vi "navX Close.vi"(8 "error in (no error)":errorcluster, 11 "navX Device TypeDef":T1={"navX Interface Protocol"=enum."SPI", "navX Interface Protocol TypeDefs"={"SPIDevRef"={"DevStatus"={"status"=FALSE, "code"=0, "source"=""}, "Handle"=0, "Controller"=enum."Controller 1", "SPI Bus"=enum."SPI On-Board, CS0"}, "I2CDevRef"={"DevStatus"={"status"=FALSE, "code"=0, "source"=""}, "Controller"=enum."Controller 1", "Device Address"=0, "Handle"=0, "I2C Bus"=enum."Invalid"}}, "navX System Information"={"Board Information"={"WhoAmI (50 | 0x32)"=0, "Board Revision"=0, "Firmware Major Version"=0, "Firmware Minor Version"=0}, "Status"={"Update Rate Hz"=0, "Accelerometer Full-Scale Range"=0, "Gyro Full-Scale Range"=0, "NAVX_OP_STATUS"=0, "NAVX_CAL_STATUS"=0, "NAVX_SELFTEST_STATUS"=0, "NAVX_SENSOR_STATUS"={"MOVING"=FALSE, "YAW_STABLE"=FALSE, "MAG_DISTURBANCE"=FALSE, "ALTITUDE_VALID"=FALSE, "SEALEVEL_PRESS_SET"=FALSE, "FUSED_HEADING_VALID"=FALSE}}, "Offsets"={"Yaw"=0.0, "Quat W"=0.0, "Quat X"=0.0, "Quat Y"=0.0, "Quat Z"=0.0}}, "navX Common Information"={"Update Rate (4Hz-60Hz)"=50, "refnum name"="", "error"={"status"=FALSE, "code"=0, "source"=""}}} {"navX Common Information"."Update Rate (4Hz-60Hz)" min=4 max=50 step=1; "navX System Information"."Status"."NAVX_OP_STATUS" items=["INITIALIZING", "SELFTEST_IN_PROGRESS", "ERROR", "IMU_AUTOCAL_IN_PROGRESS", "NORMAL"]; "navX System Information"."Status"."NAVX_CAL_STATUS" items=["IMU_CAL_STATE_MASK"=3, "IMU_CAL_INPROGRESS"=0, "IMU_CAL_ACCUMULATE"=1, "IMU_CAL_COMPLETE"=2, "MAG_CAL_COMPLETE"=4, "BARO_CAL_COMPLETE"=8]; "navX Interface Protocol TypeDefs"."I2CDevRef"."Device Address" format="%.0x"}) -> (0 "error out":errorcluster)   [LabVIEW 2014, in "navX-MXP IMU.lvlib"]
uses:
  navx-mxp_NEW/roborio/labview/navX-MXP Library/navX-MXP IMU.lvlib
  navx-mxp_NEW/roborio/labview/navX-MXP Library/COMMON/TypeDefs/navX Device TypeDef.ctl
  navx-mxp_NEW/roborio/labview/navX-MXP Library/COMMON/TypeDefs/Value TypeDefs/navX Interface Protocol.ctl
  <vilib>/Rock Robotics/WPI/SPI/WPI_SPIDevRef.ctl
  <vilib>/Rock Robotics/SystemInterfaces/Typedef/FPGA_TypedefDigitalModule.ctl
  <vilib>/Rock Robotics/SystemInterfaces/spilib/spi_bus.ctl
  <vilib>/Rock Robotics/WPI/I2C/WPI_I2CDevRef.ctl
  <vilib>/Rock Robotics/SystemInterfaces/i2clib/i2c_bus.ctl
  navx-mxp_NEW/roborio/labview/navX-MXP Library/COMMON/TypeDefs/Data TypeDefs/navX Board Information.ctl
  navx-mxp_NEW/roborio/labview/navX-MXP Library/COMMON/TypeDefs/Data TypeDefs/navX Status Data.ctl
  navx-mxp_NEW/roborio/labview/navX-MXP Library/COMMON/TypeDefs/Value TypeDefs/navX NAVX_OP_STATUS.ctl
  navx-mxp_NEW/roborio/labview/navX-MXP Library/COMMON/TypeDefs/Value TypeDefs/navX NAVX_CAL_STATUS.ctl
  navx-mxp_NEW/roborio/labview/navX-MXP Library/COMMON/TypeDefs/Value TypeDefs/navX NAVX_SENSOR_STATUS.ctl
  navx-mxp_NEW/roborio/labview/navX-MXP Library/COMMON/TypeDefs/Data TypeDefs/navX Offsets Data.ctl
  navx-mxp_NEW/roborio/labview/navX-MXP Library/COMMON/TypeDefs/Value TypeDefs/navX Update Rate.ctl
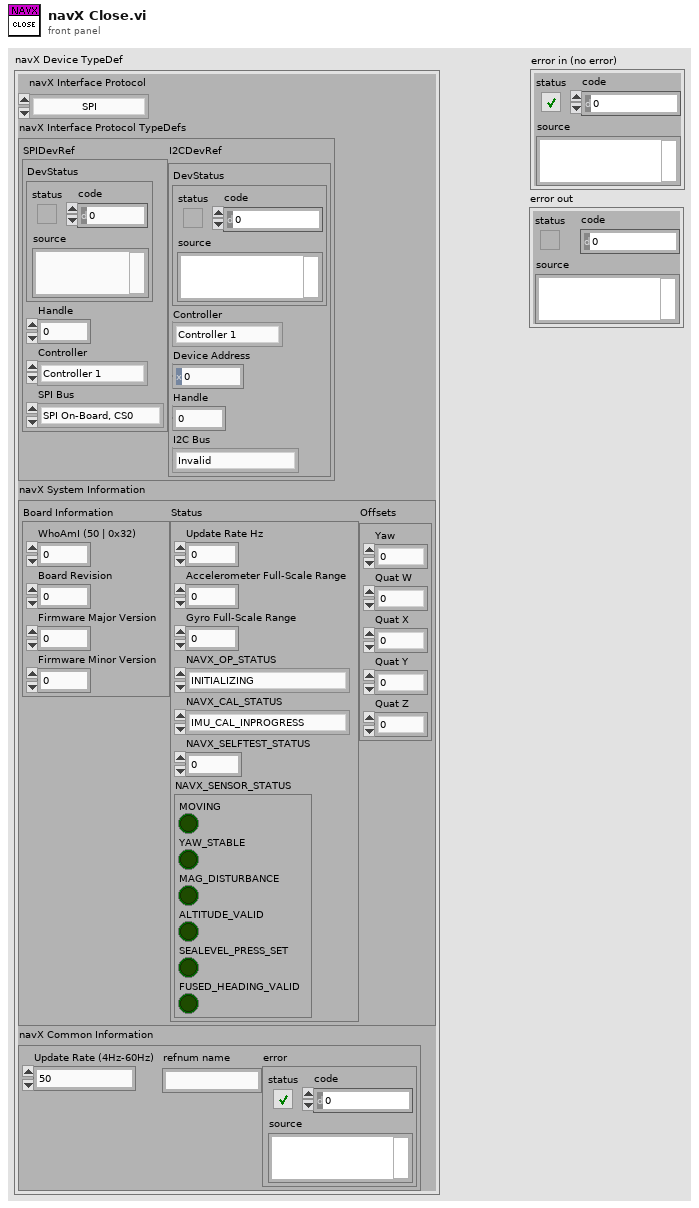
[diagram p1: front panel]
types:
  T1 = typedef "navX-MXP IMU.lvlib/navX Device TypeDef.ctl" = cluster{"navX Interface Protocol":T2, "navX Interface Protocol TypeDefs":cluster{"SPIDevRef":T3, "I2CDevRef":T6}, "navX System Information":cluster{"Board Information":T8, "Status":T9, "Offsets":T13}, "navX Common Information":cluster{"Update Rate (4Hz-60Hz)":T14, "refnum name":string, "error":errorcluster}}
  T2 = typedef "navX-MXP IMU.lvlib/navX Interface Protocol.ctl" = enum16{"SPI", "I2C"}
  T3 = typedef "WPI_SPIDevRef.ctl" = cluster{"DevStatus":errorcluster, "Handle":i32, "Controller":T4, "SPI Bus":T5}
  T4 = typedef "FPGA_TypedefDigitalModule.ctl" = enum16{"Controller 1"}
  T5 = typedef "spi_bus.ctl" = enum16{"SPI On-Board, CS0", "SPI On-Board, CS1", "SPI On-Board, CS2", "SPI On-Board, CS3", "SPI MXP", "Invalid"}
  T6 = typedef "WPI_I2CDevRef.ctl" = cluster{"DevStatus":errorcluster, "Controller":T4, "Device Address":u8, "Handle":i32, "I2C Bus":T7}
  T7 = typedef "i2c_bus.ctl" = enum16{"I2C On-Board", "I2C MXP", "Invalid"}
  T8 = typedef "navX-MXP IMU.lvlib/navX Board Information.ctl" = cluster{"WhoAmI (50 | 0x32)":u8, "Board Revision":u8, "Firmware Major Version":u8, "Firmware Minor Version":u8}
  T9 = typedef "navX-MXP IMU.lvlib/navX Status Data.ctl" = cluster{"Update Rate Hz":u8, "Accelerometer Full-Scale Range":u8, "Gyro Full-Scale Range":u16, "NAVX_OP_STATUS":T10, "NAVX_CAL_STATUS":T11, "NAVX_SELFTEST_STATUS":u8, "NAVX_SENSOR_STATUS":T12}
  T10 = typedef "navX-MXP IMU.lvlib/navX NAVX_OP_STATUS.ctl" = u8
  T11 = typedef "navX-MXP IMU.lvlib/navX NAVX_CAL_STATUS.ctl" = u8
  T12 = typedef "navX-MXP IMU.lvlib/navX NAVX_SENSOR_STATUS.ctl" = cluster{"MOVING":bool, "YAW_STABLE":bool, "MAG_DISTURBANCE":bool, "ALTITUDE_VALID":bool, "SEALEVEL_PRESS_SET":bool, "FUSED_HEADING_VALID":bool}
  T13 = typedef "navX-MXP IMU.lvlib/navX Offsets Data.ctl" = cluster{"Yaw":dbl, "Quat W":dbl, "Quat X":dbl, "Quat Y":dbl, "Quat Z":dbl}
  T14 = typedef "navX-MXP IMU.lvlib/navX Update Rate.ctl" = u8
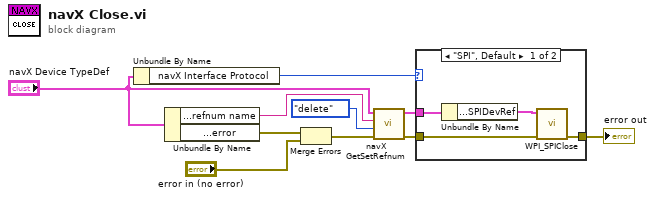
[diagram p0: block diagram]
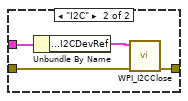
[diagram p2: hidden frame]
diagram:
  n1 = Unbundle By Name("navX Device TypeDef") -> ("navX Interface Protocol"=w4:T2)
  n2 = Unbundle By Name("navX Device TypeDef") -> ("navX Common Information.refnum name"=w10:string, "navX Common Information.error"=w8:errorcluster)
  n3 = Merge Errors(w8, "error in (no error)") -> (w7:errorcluster)
  n4 = call "navX GetSetRefnum.vi"("error in (no error)"=w7, "menu"=enum16{"set", "get", "delete"}."delete", "refnum name"=w10, "navX Device TypeDef"="navX Device TypeDef") -> ("error out"=w2:errorcluster, "navX Device TypeDef"=w5:T1)  [unwired: 6 in]
  n5 = case shown="\"SPI\", Default" w4 {
    tunnel: w5 -> [w14 w18]
    tunnel: w2 -> [w12 w16]
    tunnel: [w11 w15] -> w1
    frame "SPI", Default {
      n6 = Unbundle By Name(w14) -> ("navX Interface Protocol TypeDefs.SPIDevRef"=w13:T3)
      n7 = call <vilib>:"WPI_SPIClose.vi"("error in (no error)"=w12, "SPIDevRef"=w13) -> ("error out"=w11:errorcluster)  [unwired: 9 in]
    }
    frame "I2C" {
      n8 = Unbundle By Name(w18) -> ("navX Interface Protocol TypeDefs.I2CDevRef"=w17:T6)
      n9 = call <vilib>:"WPI_I2CClose.vi"("error in (no error)"=w16, "I2CDevRef"=w17) -> ("error out"=w15:errorcluster)  [unwired: 9 in]
    }
  }
  "error out" <- w1
